vi "Juk3boxOS.vi"   [LabVIEW 2016]
uses:
  <vilib>/NXT/Block Support/NXT_InputPort.ctl
  <vilib>/NXT/Block Support/NXT_OutputPort.ctl
  <vilib>/NXT/Block Support/NXT_ButtonSelector.ctl
  <vilib>/NXT/Dual Mode Library/Sensors/EV3_Color_Color.vi
  <vilib>/NXT/Dual Mode Library/Display/drawText.vi
  <vilib>/NXT/Dual Mode Library/Sensors/readNXTButton.vi
  <vilib>/NXT/NXTIO Xnodes/NXTIONodeSubVIs/NXTMoveMotors.vi
  <vilib>/NXT/Dual Mode Library/Waits/Wait_Num.vi
  <vilib>/NXT/NXTIO Xnodes/NXTIONodeSubVIs/NXTStopMotors.vi
  <vilib>/NXT/Dual Mode Library/Display/clearDisplay.vi
  <vilib>/NXT/Dual Mode Library/Sensors/Touch_Pressed.vi
  <vilib>/NXT/NXTIO Xnodes/AddressXNode/NXTIOAddress.xnode
  <vilib>/NXT/NXTIO Xnodes/NXTIOXNode/NXTIO.xnode
  <vilib>/NXT/Subs/LVHSConnector.ctl
  <vilib>/NXT/LegoClasses/BrickReference/BrickReference.lvclass
types:
  T1 = typedef "NXT_InputPort.ctl" = u32
  T2 = typedef "LVHSConnector.ctl" = refnum<class "BrickReference.lvclass">
  T3 = typedef "ColorSensorColors.ctl" = enum16{"No Color", "Black", "Blue", "Green", "Yellow", "Red", "White", "Brown"}
  T4 = typedef "NXT_OutputPort.ctl" = u8
  T5 = typedef "NXT_ButtonSelector.ctl" = u16
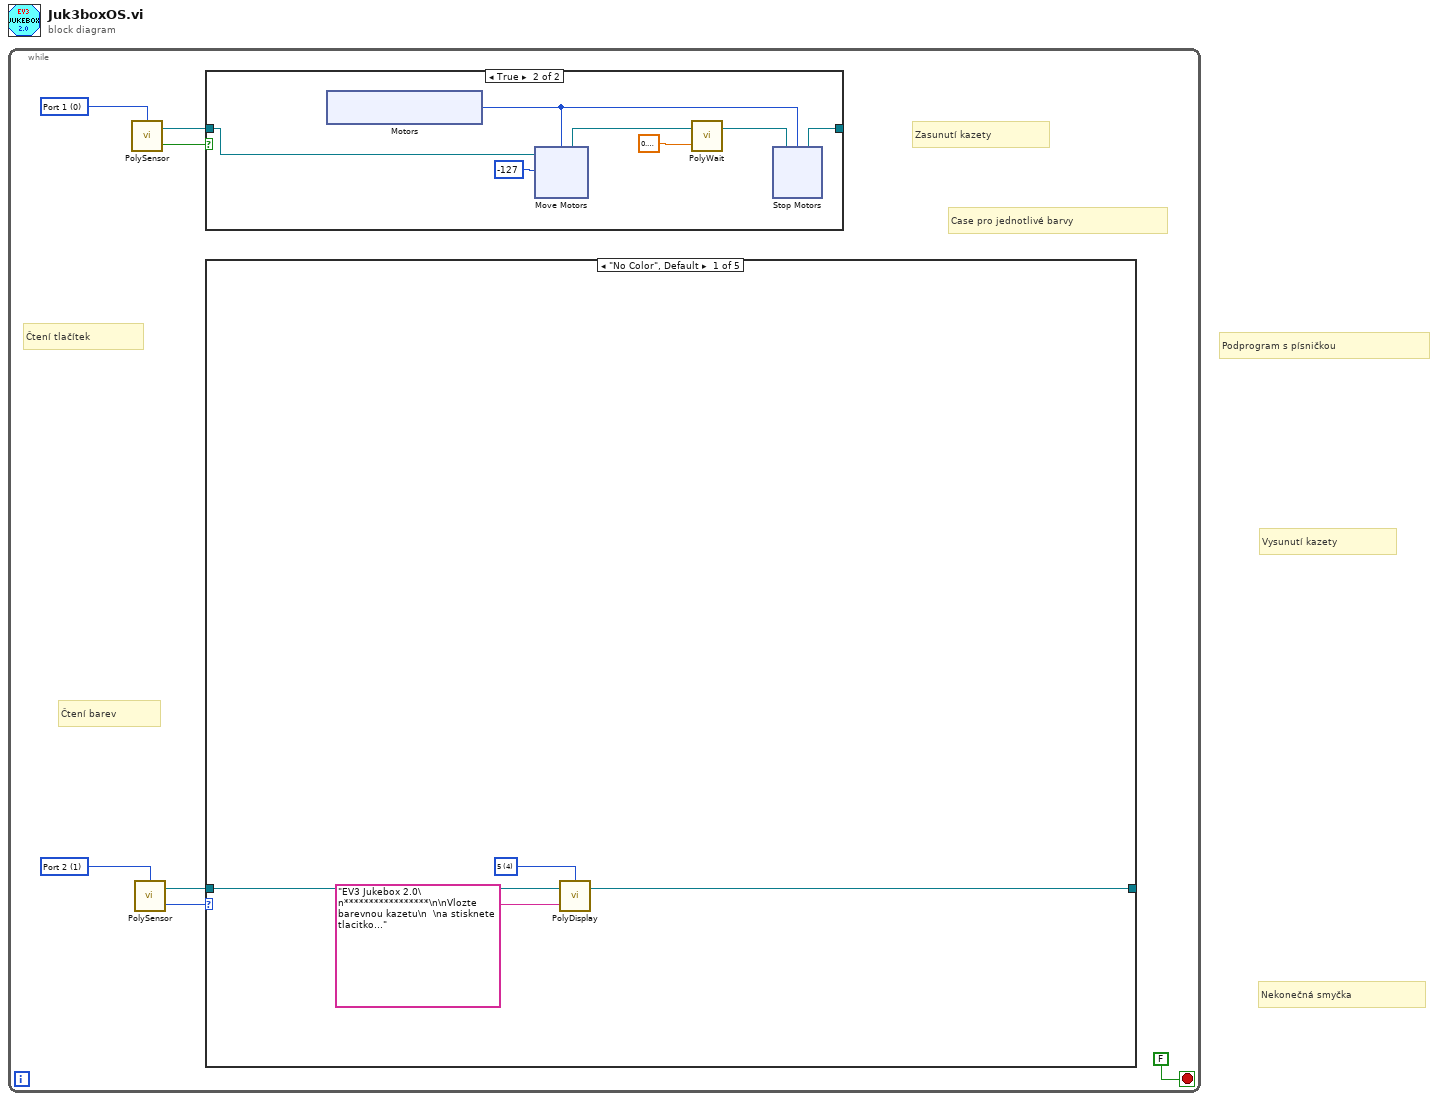
[diagram p0: block diagram]
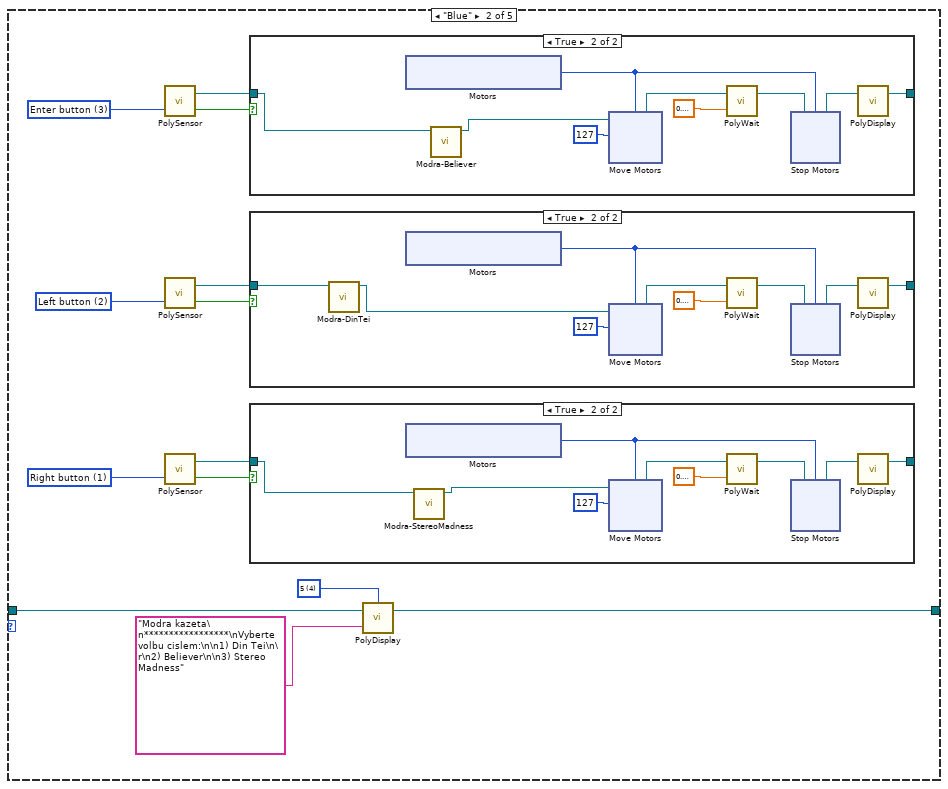
[diagram p3: hidden frame]
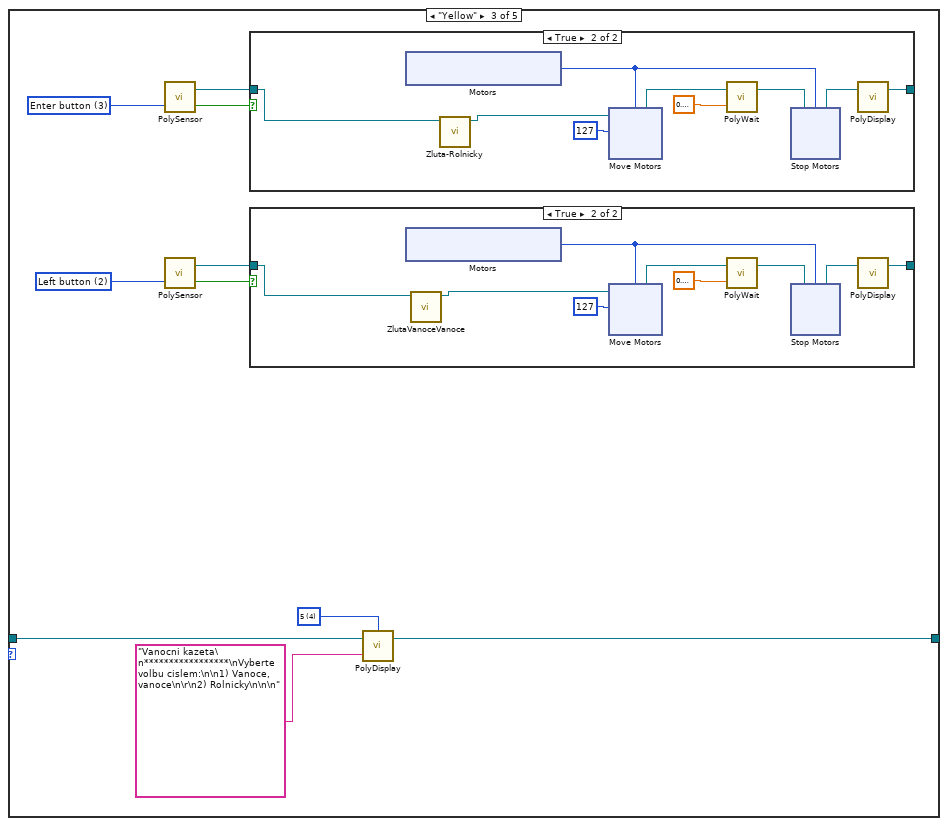
[diagram p7: hidden frame]
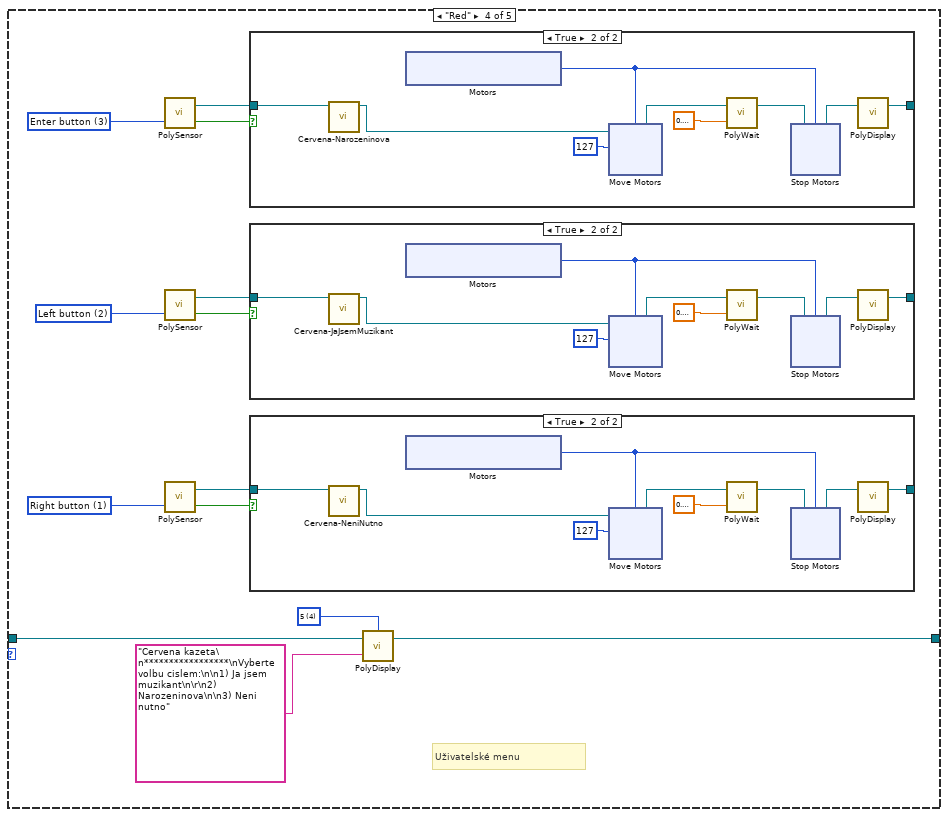
[diagram p10: hidden frame]
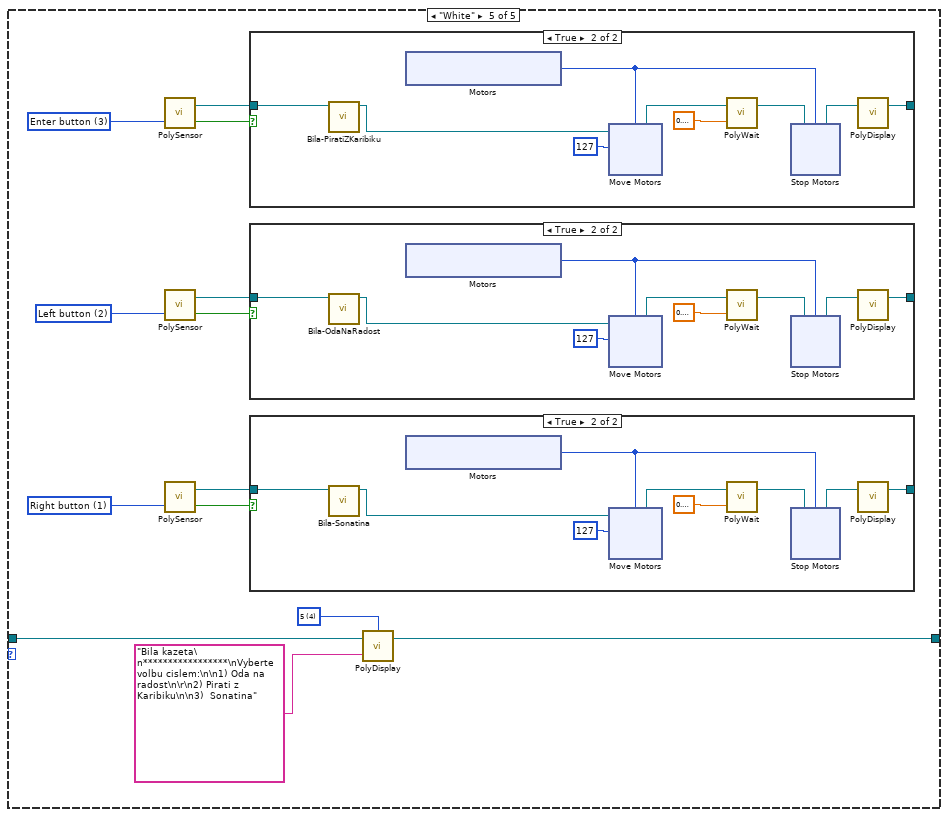
[diagram p14: hidden frame]
diagram:
  # "Nekonečná smyčka"
  # "Vysunutí kazety"
  # "Podprogram s písničkou"
  n1 = while {
    stop <- FALSE stop-if-true
    w1 = T1 0 items=["Port 1", "Port 2", "Port 3", "Port 4"] ("Port (Port 1)")
    w6 = T1 1 items=["Port 1", "Port 2", "Port 3", "Port 4"] ("Port (Port 3)")
    # "Case pro jednotlivé barvy"
    # "Čtení barev"
    # "Zasunutí kazety"
    # "Čtení tlačítek"
    n2 = call-poly <vilib>:"PolySensor.vi"("Port (Port 1)"=w1) -> ("Yes / No"=w3:bool, "NXT/EV3"=w2:T2)  [unwired: 2 in]
    n3 = call-poly <vilib>:"PolySensor.vi"("Port (Port 1)"=w6) -> ("Detected Color"=w7:T3, "NXT/EV3"=w5:T2)  [unwired: 2 in]
    n4 = case shown="True" w3 {
      tunnel: w2 -> [w8 w10]
      tunnel: [w8 w9] -> _
      frame False {
      }
      frame True {
        n5 = xnode "Motors"() -> ("Motor"=w11:T4)
        n6 = xnode "Move Motors"("Power/Speed 1"=i8 -127, "Motors"=w11, "NXT/EV3"=w10) -> ("NXT/EV3"=w14:T2)
        n7 = call-poly <vilib>:"PolyWait.vi"("Time (1 sec)"=sgl 0.7, "NXT/EV3"=w14) -> ("NXT/EV3"=w12:T2)  [unwired: 2 in]
        n8 = xnode "Stop Motors"("Motors"=w11, "NXT/EV3"=w12) -> ("NXT/EV3"=w9:T2)
      }
    }
    n9 = case shown="\"No Color\", Default" w7 {
      tunnel: w5 -> [w29 w34 w117 w172 w254]
      tunnel: [w30 w33 w116 w171 w253] -> _
      frame "No Color", Default {
        w32 = i16 4 items=["1", "2", "3", "4", "5", "6", "7", "8", "9", "10", "11", "12"] ("Line")
        n10 = call-poly <vilib>:"PolyDisplay.vi"("Text"="EV3 Jukebox 2.0\n*****************\n\nVlozte barevnou kazetu\n  \na stisknete tlacitko...", "NXT/EV3"=w29, "Line"=w32) -> ("NXT/EV3"=w30:T2)  [unwired: 1 in]
      }
      frame "Blue" {
        w38 = T5 1 items=["Enter button"=3, "Left button"=2, "Right button"=1, "Up Button"=4, "Down Button"=5] ("Button (Enter button)")
        w41 = T5 2 items=["Enter button"=3, "Left button"=2, "Right button"=1, "Up Button"=4, "Down Button"=5] ("Button (Enter button)")
        w42 = T5 3 items=["Enter button"=3, "Left button"=2, "Right button"=1, "Up Button"=4, "Down Button"=5] ("Button (Enter button)")
        w45 = i16 4 items=["1", "2", "3", "4", "5", "6", "7", "8", "9", "10", "11", "12"] ("Line")
        n11 = call-poly <vilib>:"PolySensor.vi"("Button (Enter button)"=w42) -> ("Yes/No"=w35:bool, "NXT/EV3"=w43:T2)  [unwired: 2 in]
        n12 = call-poly <vilib>:"PolySensor.vi"("Button (Enter button)"=w41) -> ("Yes/No"=w36:bool, "NXT/EV3"=w40:T2)  [unwired: 2 in]
        n13 = call-poly <vilib>:"PolySensor.vi"("Button (Enter button)"=w38) -> ("Yes/No"=w37:bool, "NXT/EV3"=w39:T2)  [unwired: 2 in]
        n14 = case shown="True" w35 {
          tunnel: w43 -> [w92 w94]
          tunnel: [w92 w98] -> _
          frame False {
          }
          frame True {
            n15 = xnode "Motors"() -> ("Motor"=w95:T4)
            n16 = call "Modra-Believer.vi"("NXT/EV3"=w94) -> ("NXT/EV3 2"=w93:T2)  [unwired: 10 in]
            n17 = xnode "Move Motors"("Power/Speed 1"=i8 127, "Motors"=w95, "NXT/EV3"=w93) -> ("NXT/EV3"=w100:T2)
            n18 = call-poly <vilib>:"PolyWait.vi"("Time (1 sec)"=sgl 0.7, "NXT/EV3"=w100) -> ("NXT/EV3"=w97:T2)  [unwired: 2 in]
            n19 = xnode "Stop Motors"("Motors"=w95, "NXT/EV3"=w97) -> ("NXT/EV3"=w96:T2)
            n20 = call-poly <vilib>:"PolyDisplay.vi"("NXT/EV3"=w96) -> ("NXT/EV3"=w98:T2)  [unwired: 3 in]
          }
        }
        n21 = case shown="True" w36 {
          tunnel: w40 -> [w69 w71]
          tunnel: [w69 w76] -> _
          frame False {
          }
          frame True {
            n22 = call "Modra-DinTei.vi"("NXT/EV3"=w71) -> ("NXT/EV3 2"=w70:T2)  [unwired: 10 in]
            n23 = xnode "Motors"() -> ("Motor"=w73:T4)
            n24 = xnode "Move Motors"("Power/Speed 1"=i8 127, "Motors"=w73, "NXT/EV3"=w70) -> ("NXT/EV3"=w78:T2)
            n25 = call-poly <vilib>:"PolyWait.vi"("Time (1 sec)"=sgl 0.7, "NXT/EV3"=w78) -> ("NXT/EV3"=w75:T2)  [unwired: 2 in]
            n26 = xnode "Stop Motors"("Motors"=w73, "NXT/EV3"=w75) -> ("NXT/EV3"=w74:T2)
            n27 = call-poly <vilib>:"PolyDisplay.vi"("NXT/EV3"=w74) -> ("NXT/EV3"=w76:T2)  [unwired: 3 in]
          }
        }
        n28 = case shown="True" w37 {
          tunnel: w39 -> [w46 w48]
          tunnel: [w46 w49] -> _
          frame False {
          }
          frame True {
            n29 = xnode "Motors"() -> ("Motor"=w50:T4)
            n30 = call "Modra-StereoMadness.vi"("NXT/EV3"=w48) -> ("NXT/EV3 2"=w47:T2)  [unwired: 10 in]
            n31 = xnode "Move Motors"("Power/Speed 1"=i8 127, "Motors"=w50, "NXT/EV3"=w47) -> ("NXT/EV3"=w54:T2)
            n32 = call-poly <vilib>:"PolyWait.vi"("Time (1 sec)"=sgl 0.7, "NXT/EV3"=w54) -> ("NXT/EV3"=w52:T2)  [unwired: 2 in]
            n33 = xnode "Stop Motors"("Motors"=w50, "NXT/EV3"=w52) -> ("NXT/EV3"=w51:T2)
            n34 = call-poly <vilib>:"PolyDisplay.vi"("NXT/EV3"=w51) -> ("NXT/EV3"=w49:T2)  [unwired: 3 in]
          }
        }
        n35 = call-poly <vilib>:"PolyDisplay.vi"("Text"="Modra kazeta\n*****************\nVyberte volbu cislem:\n\n1) Din Tei\n\r\n2) Believer\n\n3) Stereo Madness", "NXT/EV3"=w34, "Line"=w45) -> ("NXT/EV3"=w33:T2)  [unwired: 1 in]
      }
      frame "Yellow" {
        w115 = i16 4 items=["1", "2", "3", "4", "5", "6", "7", "8", "9", "10", "11", "12"] ("Line")
        w121 = T5 2 items=["Enter button"=3, "Left button"=2, "Right button"=1, "Up Button"=4, "Down Button"=5] ("Button (Enter button)")
        w122 = T5 3 items=["Enter button"=3, "Left button"=2, "Right button"=1, "Up Button"=4, "Down Button"=5] ("Button (Enter button)")
        n36 = call-poly <vilib>:"PolySensor.vi"("Button (Enter button)"=w122) -> ("Yes/No"=w118:bool, "NXT/EV3"=w123:T2)  [unwired: 2 in]
        n37 = call-poly <vilib>:"PolySensor.vi"("Button (Enter button)"=w121) -> ("Yes/No"=w119:bool, "NXT/EV3"=w120:T2)  [unwired: 2 in]
        n38 = case shown="True" w118 {
          tunnel: w123 -> [w148 w150]
          tunnel: [w148 w154] -> _
          frame False {
          }
          frame True {
            n39 = xnode "Motors"() -> ("Motor"=w151:T4)
            n40 = call "Zluta-Rolnicky.vi"("NXT/EV3"=w150) -> ("NXT/EV3 2"=w149:T2)  [unwired: 10 in]
            n41 = xnode "Move Motors"("Power/Speed 1"=i8 127, "Motors"=w151, "NXT/EV3"=w149) -> ("NXT/EV3"=w156:T2)
            n42 = call-poly <vilib>:"PolyWait.vi"("Time (1 sec)"=sgl 0.7, "NXT/EV3"=w156) -> ("NXT/EV3"=w153:T2)  [unwired: 2 in]
            n43 = xnode "Stop Motors"("Motors"=w151, "NXT/EV3"=w153) -> ("NXT/EV3"=w152:T2)
            n44 = call-poly <vilib>:"PolyDisplay.vi"("NXT/EV3"=w152) -> ("NXT/EV3"=w154:T2)  [unwired: 3 in]
          }
        }
        n45 = case shown="True" w119 {
          tunnel: w120 -> [w125 w127]
          tunnel: [w125 w132] -> _
          frame False {
          }
          frame True {
            n46 = xnode "Motors"() -> ("Motor"=w129:T4)
            n47 = call "ZlutaVanoceVanoce.vi"("NXT/EV3"=w127) -> ("NXT/EV3 2"=w126:T2)  [unwired: 10 in]
            n48 = xnode "Move Motors"("Power/Speed 1"=i8 127, "Motors"=w129, "NXT/EV3"=w126) -> ("NXT/EV3"=w134:T2)
            n49 = call-poly <vilib>:"PolyWait.vi"("Time (1 sec)"=sgl 0.7, "NXT/EV3"=w134) -> ("NXT/EV3"=w131:T2)  [unwired: 2 in]
            n50 = xnode "Stop Motors"("Motors"=w129, "NXT/EV3"=w131) -> ("NXT/EV3"=w130:T2)
            n51 = call-poly <vilib>:"PolyDisplay.vi"("NXT/EV3"=w130) -> ("NXT/EV3"=w132:T2)  [unwired: 3 in]
          }
        }
        n52 = call-poly <vilib>:"PolyDisplay.vi"("Text"="Vanocni kazeta\n*****************\nVyberte volbu cislem:\n\n1) Vanoce, vanoce\n\r\n2) Rolnicky\n\n\n", "NXT/EV3"=w117, "Line"=w115) -> ("NXT/EV3"=w116:T2)  [unwired: 1 in]
      }
      frame "Red" {
        w176 = T5 1 items=["Enter button"=3, "Left button"=2, "Right button"=1, "Up Button"=4, "Down Button"=5] ("Button (Enter button)")
        w179 = T5 2 items=["Enter button"=3, "Left button"=2, "Right button"=1, "Up Button"=4, "Down Button"=5] ("Button (Enter button)")
        w180 = T5 3 items=["Enter button"=3, "Left button"=2, "Right button"=1, "Up Button"=4, "Down Button"=5] ("Button (Enter button)")
        w183 = i16 4 items=["1", "2", "3", "4", "5", "6", "7", "8", "9", "10", "11", "12"] ("Line")
        # "Uživatelské menu"
        n53 = call-poly <vilib>:"PolySensor.vi"("Button (Enter button)"=w180) -> ("Yes/No"=w173:bool, "NXT/EV3"=w181:T2)  [unwired: 2 in]
        n54 = call-poly <vilib>:"PolySensor.vi"("Button (Enter button)"=w179) -> ("Yes/No"=w174:bool, "NXT/EV3"=w178:T2)  [unwired: 2 in]
        n55 = call-poly <vilib>:"PolySensor.vi"("Button (Enter button)"=w176) -> ("Yes/No"=w175:bool, "NXT/EV3"=w177:T2)  [unwired: 2 in]
        n56 = case shown="True" w173 {
          tunnel: w181 -> [w230 w231]
          tunnel: [w230 w235] -> _
          frame False {
          }
          frame True {
            n57 = call "Cervena-Narozeninova.vi"("NXT/EV3"=w231) -> ("NXT/EV3 2"=w236:T2)  [unwired: 10 in]
            n58 = xnode "Motors"() -> ("Motor"=w232:T4)
            n59 = xnode "Move Motors"("Power/Speed 1"=i8 127, "Motors"=w232, "NXT/EV3"=w236) -> ("NXT/EV3"=w238:T2)
            n60 = call-poly <vilib>:"PolyWait.vi"("Time (1 sec)"=sgl 0.7, "NXT/EV3"=w238) -> ("NXT/EV3"=w234:T2)  [unwired: 2 in]
            n61 = xnode "Stop Motors"("Motors"=w232, "NXT/EV3"=w234) -> ("NXT/EV3"=w233:T2)
            n62 = call-poly <vilib>:"PolyDisplay.vi"("NXT/EV3"=w233) -> ("NXT/EV3"=w235:T2)  [unwired: 3 in]
          }
        }
        n63 = case shown="True" w174 {
          tunnel: w178 -> [w207 w209]
          tunnel: [w207 w213] -> _
          frame False {
          }
          frame True {
            n64 = call "Cervena-JaJsemMuzikant .vi"("NXT/EV3"=w209) -> ("NXT/EV3 2"=w214:T2)  [unwired: 10 in]
            n65 = xnode "Motors"() -> ("Motor"=w210:T4)
            n66 = xnode "Move Motors"("Power/Speed 1"=i8 127, "Motors"=w210, "NXT/EV3"=w214) -> ("NXT/EV3"=w216:T2)
            n67 = call-poly <vilib>:"PolyWait.vi"("Time (1 sec)"=sgl 0.7, "NXT/EV3"=w216) -> ("NXT/EV3"=w212:T2)  [unwired: 2 in]
            n68 = xnode "Stop Motors"("Motors"=w210, "NXT/EV3"=w212) -> ("NXT/EV3"=w211:T2)
            n69 = call-poly <vilib>:"PolyDisplay.vi"("NXT/EV3"=w211) -> ("NXT/EV3"=w213:T2)  [unwired: 3 in]
          }
        }
        n70 = case shown="True" w175 {
          tunnel: w177 -> [w184 w187]
          tunnel: [w184 w185] -> _
          frame False {
          }
          frame True {
            n71 = call "Cervena-NeniNutno.vi"("NXT/EV3"=w187) -> ("NXT/EV3 2"=w186:T2)  [unwired: 10 in]
            n72 = xnode "Motors"() -> ("Motor"=w188:T4)
            n73 = xnode "Move Motors"("Power/Speed 1"=i8 127, "Motors"=w188, "NXT/EV3"=w186) -> ("NXT/EV3"=w192:T2)
            n74 = call-poly <vilib>:"PolyWait.vi"("Time (1 sec)"=sgl 0.7, "NXT/EV3"=w192) -> ("NXT/EV3"=w190:T2)  [unwired: 2 in]
            n75 = xnode "Stop Motors"("Motors"=w188, "NXT/EV3"=w190) -> ("NXT/EV3"=w189:T2)
            n76 = call-poly <vilib>:"PolyDisplay.vi"("NXT/EV3"=w189) -> ("NXT/EV3"=w185:T2)  [unwired: 3 in]
          }
        }
        n77 = call-poly <vilib>:"PolyDisplay.vi"("Text"="Cervena kazeta\n*****************\nVyberte volbu cislem:\n\n1) Ja jsem muzikant\n\r\n2) Narozeninova\n\n3) Neni nutno", "NXT/EV3"=w172, "Line"=w183) -> ("NXT/EV3"=w171:T2)  [unwired: 1 in]
      }
      frame "White" {
        w258 = T5 1 items=["Enter button"=3, "Left button"=2, "Right button"=1, "Up Button"=4, "Down Button"=5] ("Button (Enter button)")
        w261 = T5 2 items=["Enter button"=3, "Left button"=2, "Right button"=1, "Up Button"=4, "Down Button"=5] ("Button (Enter button)")
        w262 = T5 3 items=["Enter button"=3, "Left button"=2, "Right button"=1, "Up Button"=4, "Down Button"=5] ("Button (Enter button)")
        w265 = i16 4 items=["1", "2", "3", "4", "5", "6", "7", "8", "9", "10", "11", "12"] ("Line")
        n78 = call-poly <vilib>:"PolySensor.vi"("Button (Enter button)"=w262) -> ("Yes/No"=w255:bool, "NXT/EV3"=w263:T2)  [unwired: 2 in]
        n79 = call-poly <vilib>:"PolySensor.vi"("Button (Enter button)"=w261) -> ("Yes/No"=w256:bool, "NXT/EV3"=w260:T2)  [unwired: 2 in]
        n80 = call-poly <vilib>:"PolySensor.vi"("Button (Enter button)"=w258) -> ("Yes/No"=w257:bool, "NXT/EV3"=w259:T2)  [unwired: 2 in]
        n81 = case shown="True" w255 {
          tunnel: w263 -> [w312 w314]
          tunnel: [w312 w318] -> _
          frame False {
          }
          frame True {
            n82 = call "Bila-PiratiZKaribiku.vi"("NXT/EV3"=w314) -> ("NXT/EV3 2"=w313:T2)  [unwired: 10 in]
            n83 = xnode "Motors"() -> ("Motor"=w315:T4)
            n84 = xnode "Move Motors"("Power/Speed 1"=i8 127, "Motors"=w315, "NXT/EV3"=w313) -> ("NXT/EV3"=w320:T2)
            n85 = call-poly <vilib>:"PolyWait.vi"("Time (1 sec)"=sgl 0.7, "NXT/EV3"=w320) -> ("NXT/EV3"=w317:T2)  [unwired: 2 in]
            n86 = xnode "Stop Motors"("Motors"=w315, "NXT/EV3"=w317) -> ("NXT/EV3"=w316:T2)
            n87 = call-poly <vilib>:"PolyDisplay.vi"("NXT/EV3"=w316) -> ("NXT/EV3"=w318:T2)  [unwired: 3 in]
          }
        }
        n88 = case shown="True" w256 {
          tunnel: w260 -> [w289 w291]
          tunnel: [w289 w296] -> _
          frame False {
          }
          frame True {
            n89 = call "Bila-OdaNaRadost.vi"("NXT/EV3"=w291) -> ("NXT/EV3 2"=w290:T2)  [unwired: 10 in]
            n90 = xnode "Motors"() -> ("Motor"=w293:T4)
            n91 = xnode "Move Motors"("Power/Speed 1"=i8 127, "Motors"=w293, "NXT/EV3"=w290) -> ("NXT/EV3"=w298:T2)
            n92 = call-poly <vilib>:"PolyWait.vi"("Time (1 sec)"=sgl 0.7, "NXT/EV3"=w298) -> ("NXT/EV3"=w295:T2)  [unwired: 2 in]
            n93 = xnode "Stop Motors"("Motors"=w293, "NXT/EV3"=w295) -> ("NXT/EV3"=w294:T2)
            n94 = call-poly <vilib>:"PolyDisplay.vi"("NXT/EV3"=w294) -> ("NXT/EV3"=w296:T2)  [unwired: 3 in]
          }
        }
        n95 = case shown="True" w257 {
          tunnel: w259 -> [w266 w268]
          tunnel: [w266 w269] -> _
          frame False {
          }
          frame True {
            n96 = call "Bila-Sonatina.vi"("NXT/EV3"=w268) -> ("NXT/EV3 2"=w267:T2)  [unwired: 10 in]
            n97 = xnode "Motors"() -> ("Motor"=w270:T4)
            n98 = xnode "Move Motors"("Power/Speed 1"=i8 127, "Motors"=w270, "NXT/EV3"=w267) -> ("NXT/EV3"=w274:T2)
            n99 = call-poly <vilib>:"PolyWait.vi"("Time (1 sec)"=sgl 0.7, "NXT/EV3"=w274) -> ("NXT/EV3"=w272:T2)  [unwired: 2 in]
            n100 = xnode "Stop Motors"("Motors"=w270, "NXT/EV3"=w272) -> ("NXT/EV3"=w271:T2)
            n101 = call-poly <vilib>:"PolyDisplay.vi"("NXT/EV3"=w271) -> ("NXT/EV3"=w269:T2)  [unwired: 3 in]
          }
        }
        n102 = call-poly <vilib>:"PolyDisplay.vi"("Text"="Bila kazeta\n*****************\nVyberte volbu cislem:\n\n1) Oda na radost\n\r\n2) Pirati z Karibiku\n\n3)  Sonatina", "NXT/EV3"=w254, "Line"=w265) -> ("NXT/EV3"=w253:T2)  [unwired: 1 in]
      }
    }
  }
